vi "CMN_Read_Characters_From_File.vi"(0 "file path":path, 2 "number of characters (all:-1)":i32=-1, 3 "start of read offset (chars.:0)":i32, 5 "convert eol? (no:F)":bool) -> (6 "new file path (NotAPath if cancelled)":path, 7 "character string":string, 8 "EOF?":bool, 9 "mark after read (chars.)":i32)   [LabVIEW 2016]
doc: "LabVIEW no longer supports this VI. Use the Read Text function instead. Reads a specified number of characters from a byte stream file beginning at a specified character offset. The VI opens the file before reading from it and closes it afterwards."
panel:
  in  "prompt":string="Choose file to read."
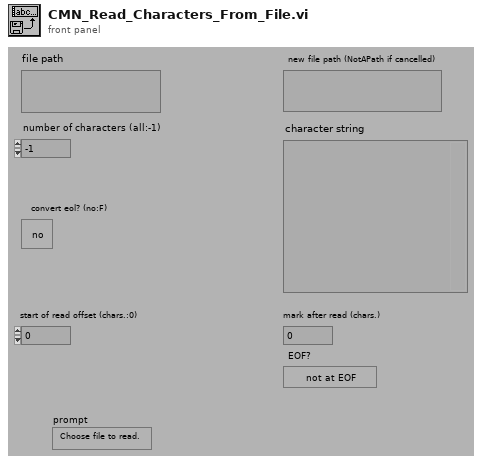
[diagram p1: front panel]
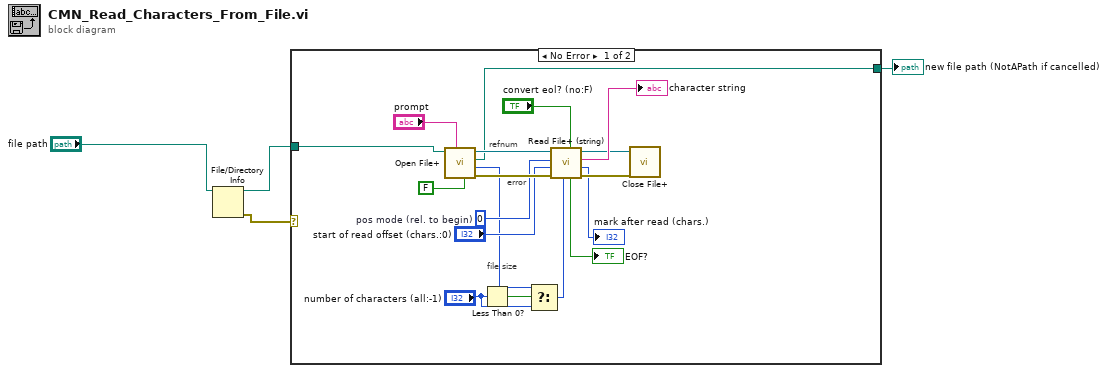
[diagram p0: block diagram]
diagram:
  n1 = File/Directory Info(path="file path") -> (path out=w3:path, error out=w4:errorcluster)  [unwired: 1 in, 5 out]
  n2 = case shown="No Error" w4 {
    tunnel: w3 -> [w22 w23]
    tunnel: [w6 w23] -> w2
    frame No Error {
      w19 = i16 0  # pos mode (rel. to begin)
      # "file size"
      # "error"
      # "refnum"
      n3 = call <vilib>:"Open File+.vi"("advisory dialog? (display:T)"=FALSE, "prompt"="prompt", "file path (\" \")"=w22) -> ("error out"=w21:errorcluster, "file size (bytes)"=w11:i32, "file path"=w6:path, "refnum"=w13:refnum<file>)  [unwired: 4 in, 1 out]
      n4 = Less Than 0?(x="number of characters (all:-1)") -> (x < 0?=w12:bool)
      n5 = Select(t=w11, s=w12, f="number of characters (all:-1)") -> (s? t:f=w9:i32)
      n6 = call <vilib>:"Read File+ (string).vi"("convert eol? (no:F)"="convert eol? (no:F)", "count"=w9, "error in (no error)"=w21, "pos offset (bytes:0)"="start of read offset (chars.:0)", "pos mode (rel. to current:2)"=w19, "refnum"=w13) -> ("error out"=w17:errorcluster, "mark after read (bytes)"=→"mark after read (chars.)":i32, "string"=→"character string":string, "dup refnum"=w16:refnum<file>, "EOF?"=→"EOF?":bool)  [unwired: 1 out]
      n7 = call <vilib>:"Close File+.vi"("error in (no error)"=w17, "refnum"=w16) -> ()  [unwired: 6 out]
    }
    frame Error {
    }
  }
  "new file path (NotAPath if cancelled)" <- w2
